vi "Write RunNotifier.vi"(8 "error in (no error)":errorcluster, 10 "RunNotifier":refnum<notifier>, 11 "O3 Frequency Train Actor in":refnum<class "O3 Frequency Train Actor.lvclass">) -> (0 "error out":errorcluster, 3 "O3 Frequency Train Actor out":refnum<class "O3 Frequency Train Actor.lvclass">)   [LabVIEW 2014, in "Calibration.lvlib" / "O3 Frequency Train Actor.lvclass"]
uses:
  O3 Frequency Train Actor.lvclass
  O3 Frequency Train Actor.lvclass/O3 Frequency Train Actor.ctl
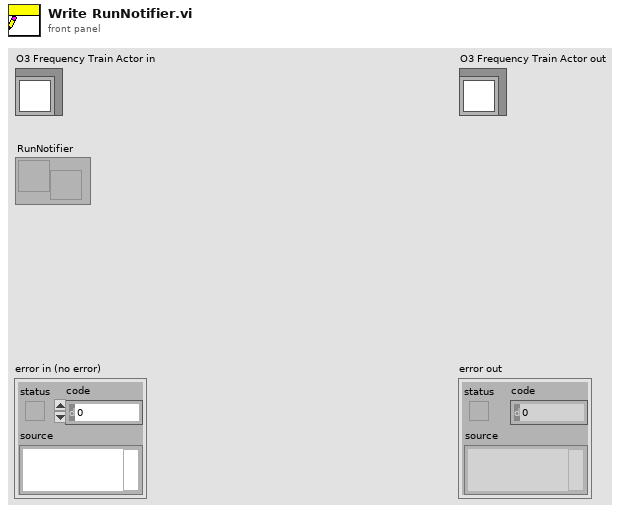
[diagram p1: front panel]
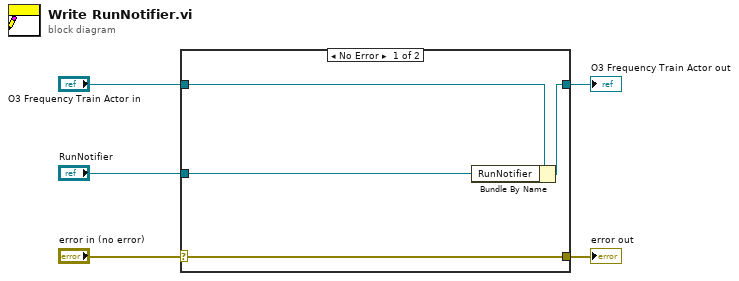
[diagram p0: block diagram]
diagram:
  n1 = case shown="No Error" "error in (no error)" {
    selector: "error in (no error)" -> [w9 w10]
    tunnel: [w9 w10] -> w4
    tunnel: [w7 w11] -> w2
    tunnel: "O3 Frequency Train Actor in" -> [w8 w11]
    tunnel: "RunNotifier" -> [w6 _]
    frame No Error {
      n2 = Bundle By Name(cluster=w8, "RunNotifier"=w6) -> (w7:refnum<class "O3 Frequency Train Actor.lvclass">)
    }
    frame Error {
    }
  }
  "error out" <- w4
  "O3 Frequency Train Actor out" <- w2
